vi "initializer_save_spec.vi"(9 "# Lines":i32, 10 "Spec File Loaded?":refnum<vi>, 11 "Parameters Tree":refnum<vi>) -> ()   [LabVIEW 2019]
uses:
  lib/libSpecValiReader.so
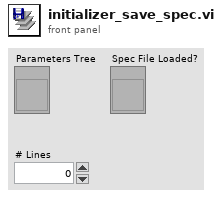
[diagram p1: front panel]
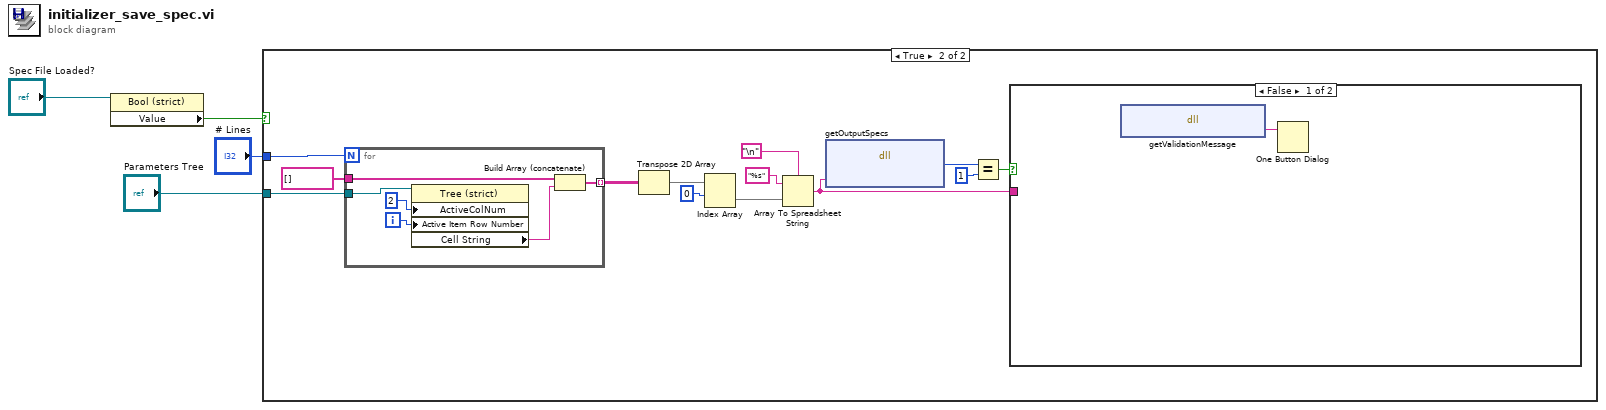
[diagram p0: block diagram]
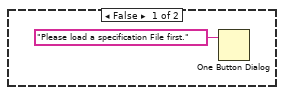
[diagram p2: hidden frame]
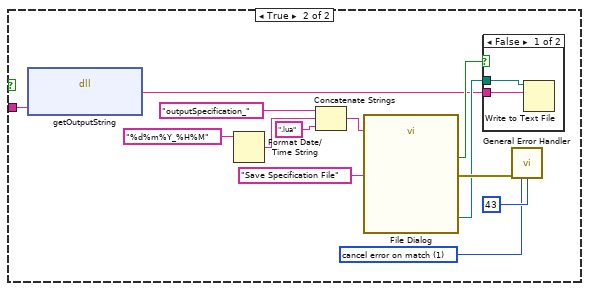
[diagram p3: hidden frame]
diagram:
  n1 = property class="Bool (strict)"(reference="Spec File Loaded?") -> ("Value"=w1:bool)  [unwired: 1 in, 2 out]
  n2 = case shown="True" w1 {
    tunnel: "# Lines" -> [_ w9]
    tunnel: "Parameters Tree" -> [_ w6]
    frame False {
      n3 = One Button Dialog(message="Please load a specification File first.") -> ()  [unwired: 1 in, 1 out]
    }
    frame True {
      n4 = for {
        N: w9 -> [_]
        tunnel: string[] [] ("Empty Val Arr") -> [w22]
        tunnel: [w21] -> w17 mode=indexing
        tunnel: w6 -> [w19]
        i -> [w24]
        n5 = property on="Property Node" class="Tree (strict)"(reference=w19, "ActiveColNum"=2 ("Active Cell:Active Column Number"), "Active Item Row Number"=w24) -> ("Cell String"=w20:string)  [unwired: 1 in, 2 out]
        n6 = Build Array (concatenate)(w22, w20) -> (w21:string[])
      }
      n7 = Transpose 2D Array(2D array=w17) -> (transposed array=w16:string[][])
      n8 = Index Array(array=w16, index (row)=0) -> (element=w15:string[])  [unwired: 1 in]
      n9 = Array To Spreadsheet String(delimiter (Tab)="\n", array=w15, 3:"%s" ("format string")) -> (spreadsheet string=w7:string)
      n10 = dll-call lib="home/paul/Schreibtisch/Biogas_plant_setup/lib/libSpecValiReader.so" fn="getOutputSpecs"("inputSpecs"=w7) -> ("isValid"=w8:i32)  [unwired: 4 in, 2 out]
      n11 = Equal?(x=w8, y=1) -> (x = y?=w11:bool)
      n12 = case shown="False" w11 {
        tunnel: w7 -> [_ w38]
        frame False {
          n13 = dll-call lib="home/paul/Schreibtisch/Biogas_plant_setup/lib/libSpecValiReader.so" fn="getValidationMessage"() -> ("validationMessage"=w25:string)  [unwired: 3 in, 2 out]
          n14 = One Button Dialog(message=w25) -> ()  [unwired: 1 in, 1 out]
        }
        frame True {
          w33 = 1 items=["no exception", "cancel error on match", "set error on match"] ("[exception action] (none:0)")
          n15 = dll-call lib="home/paul/Schreibtisch/Biogas_plant_setup/lib/libSpecValiReader.so" fn="getOutputString"("inputSpecs"=w38) -> ("outputString"=w31:string)  [unwired: 4 in, 2 out]
          n16 = Format Date/Time String(time format string (%c)="%d%m%Y_%H%M") -> (date/time string=w27:string)  [unwired: 2 in]
          n17 = Concatenate Strings("outputSpecification_" ("string"), w27, ".lua" ("string")) -> (w29:string)
          n18 = call "File Dialog"("prompt"="Save Specification File", "default name"=w29) -> ("selected path"=w32:path, "cancelled"=w36:bool, "error out"=w35:errorcluster)  [unwired: 10 in, 1 out]
          n19 = case shown="False" w36 {
            tunnel: w32 -> [w40 _]
            tunnel: w31 -> [w39 _]
            frame False {
              n20 = Write to Text File(file (use dialog)=w40, text=w39) -> ()  [unwired: 2 in, 3 out]
            }
            frame True {
            }
          }
          n21 = call <vilib>:"General Error Handler.vi"("error in (no error)"=w35, "[exception action] (none:0)"=w33, "[exception code]"=43) -> ()  [unwired: 8 in, 5 out]
        }
      }
    }
  }
